vi "VisualizeLog.vi"() -> ()   [LabVIEW 2018, in "Visualization.lvlib" / "VisualizeStatus.lvclass"]
doc: "This VI opens the error log on file and displays all errors that have been logged to file."
uses:
  VisualizeStatus.lvclass
  VisualizeBase/VisualizeBase_class/Requests/clUserEventType.ctl
  <vilib>/event_ctls.llb/usereventprio.ctl
  <vilib>/Utility/error.llb/Error Cluster From Error Code.vi
  <vilib>/ErrorRing/Error Ring.xnode
  VisualizeBase/VisualizeBase_class/VisualizeBase.lvclass
  <userlib>/NIST/NISTErrorLib/NISTErrorLib.lvlib
panel:
  in  "btnClearFile":bool
  in  "btnClear":bool
  out "error out":errorcluster
  in  "File Path Control":path
  out "Status Message":string
  in  "btnRefresh":bool
  in  "QueName":string="ErrorLogVisQue"
  out "ErrorArray":errorcluster[](array[cluster])
  in  "btnStop":bool
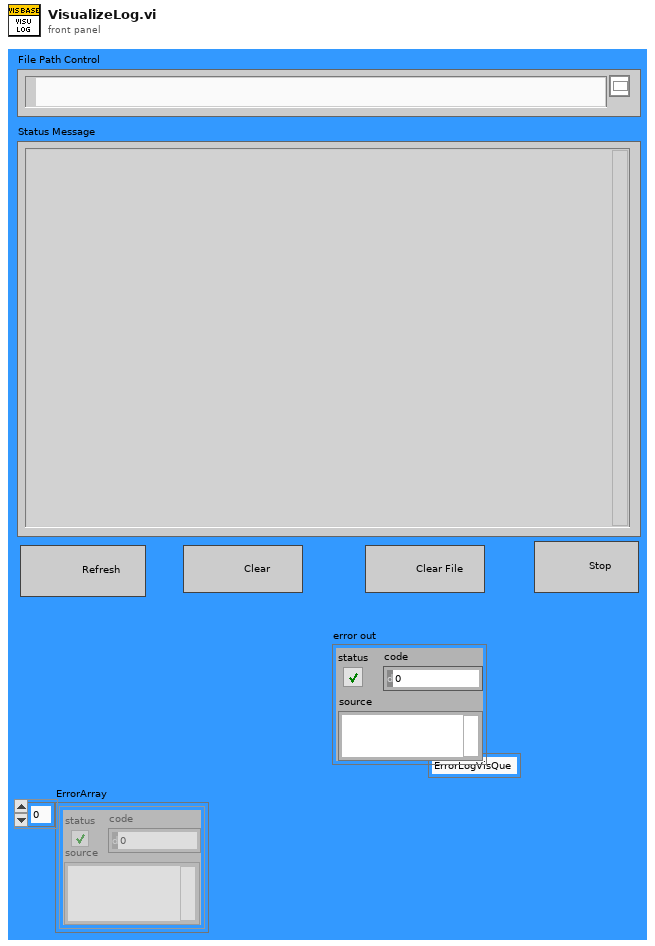
[diagram p1: front panel]
types:
  T1 = typedef "Visualization.lvlib/VisualizeBase.lvclass/clRequestEvents.ctl" = cluster{"StopRequest":refnum<user-event>, "ResetRequest":refnum<user-event>}
  T2 = enum16{"open", "replace", "create", "open or create", "replace or create", "replace or create with confirmation"}
  T3 = typedef "usereventprio.ctl" = enum32{"high priority", "normal priority"}
  T4 = typedef "Visualization.lvlib/VisualizeBase.lvclass/clUserEventType.ctl" = cluster{"BusIndex":i8, "Data":variant}
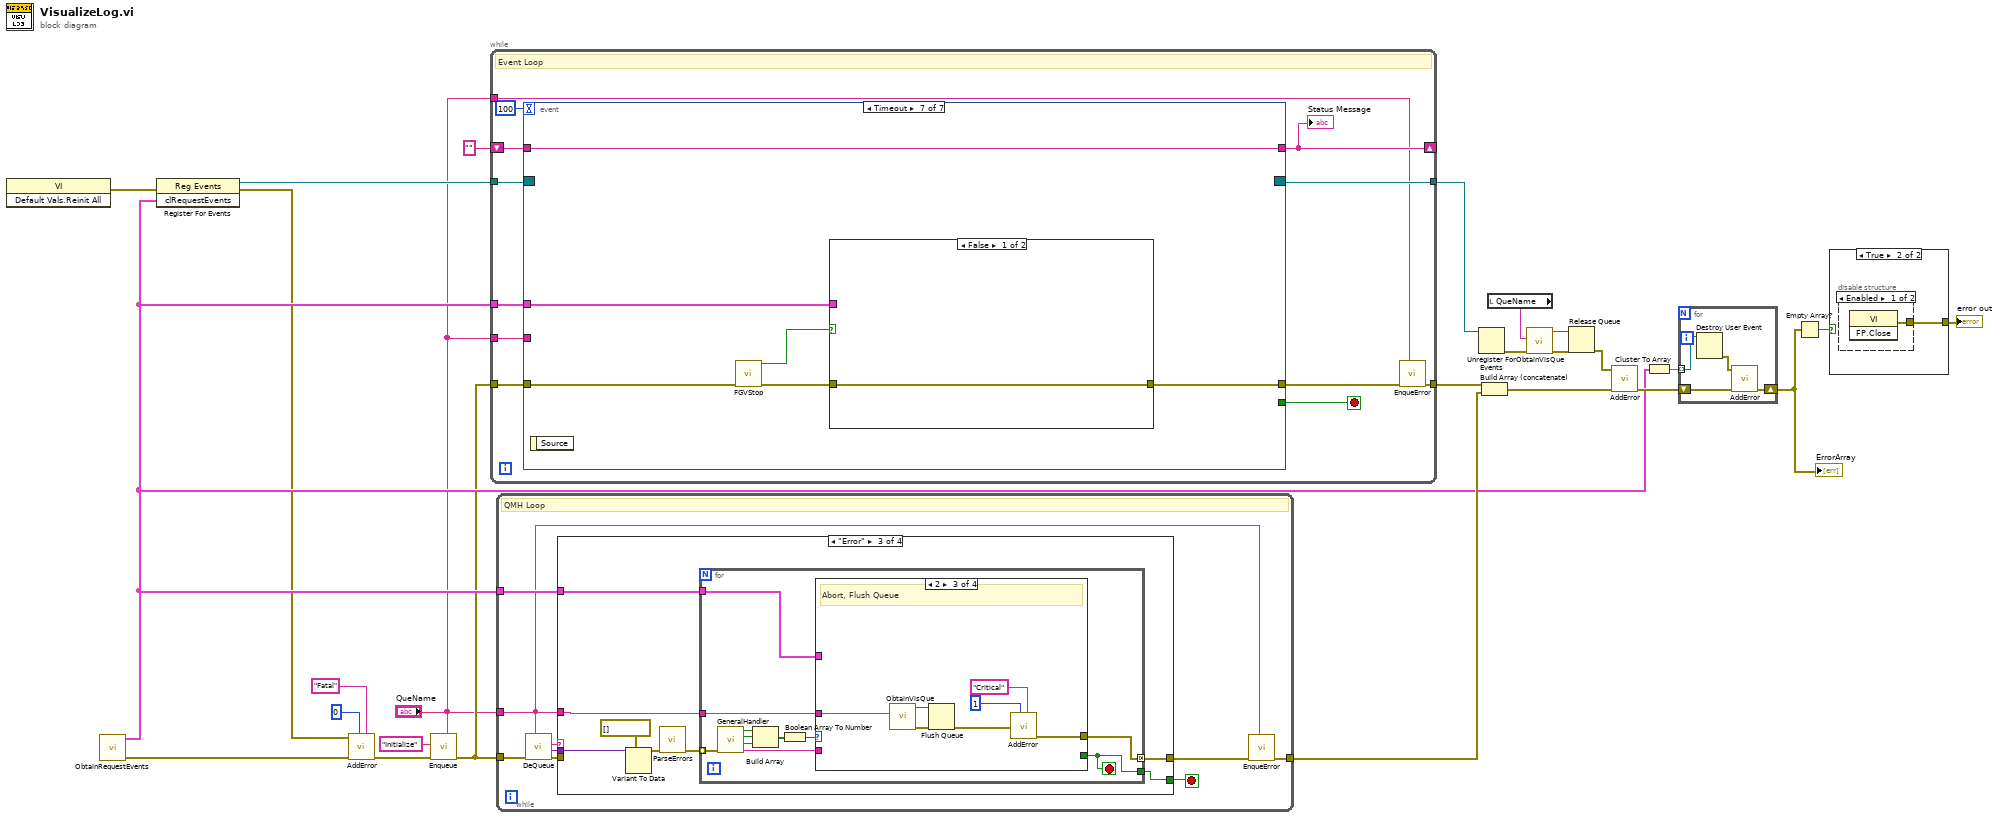
[diagram p0: block diagram]
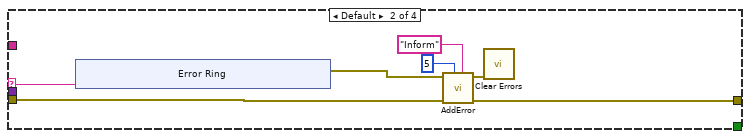
[diagram p3: hidden frame]
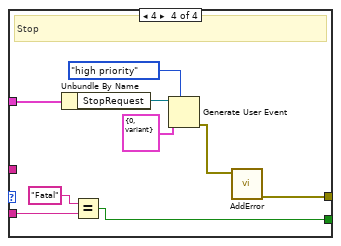
[diagram p6: hidden frame]
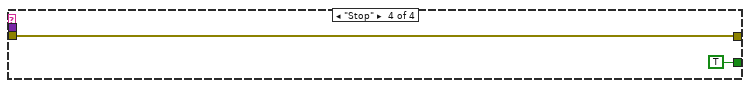
[diagram p7: hidden frame]
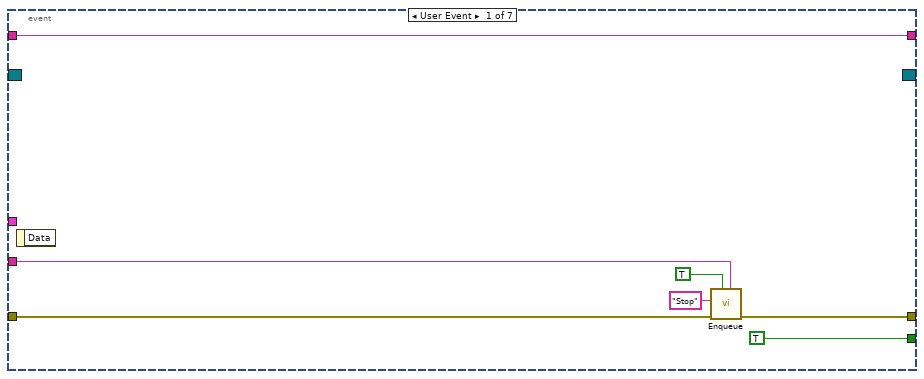
[diagram p8: hidden frame]
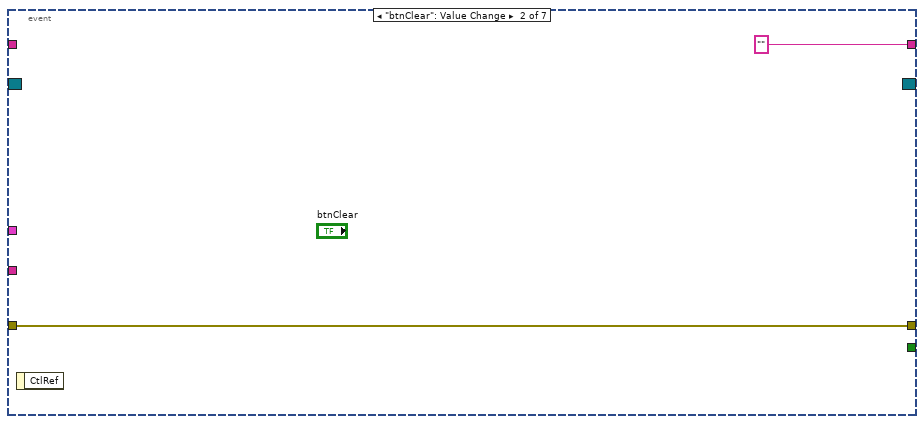
[diagram p9: hidden frame]
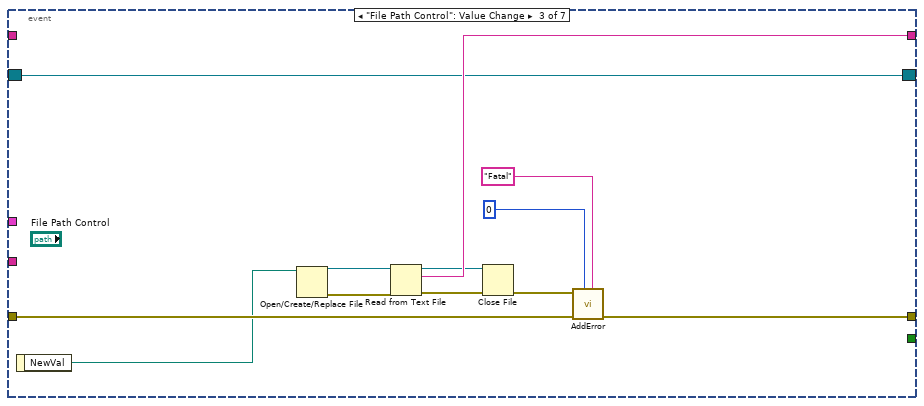
[diagram p10: hidden frame]
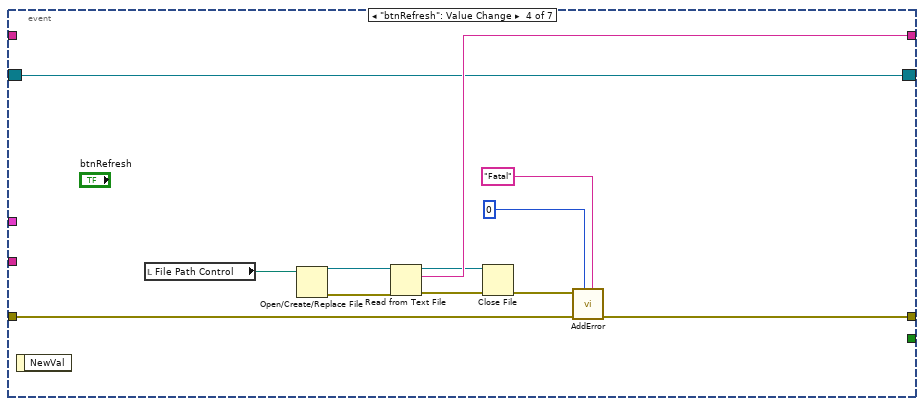
[diagram p11: hidden frame]
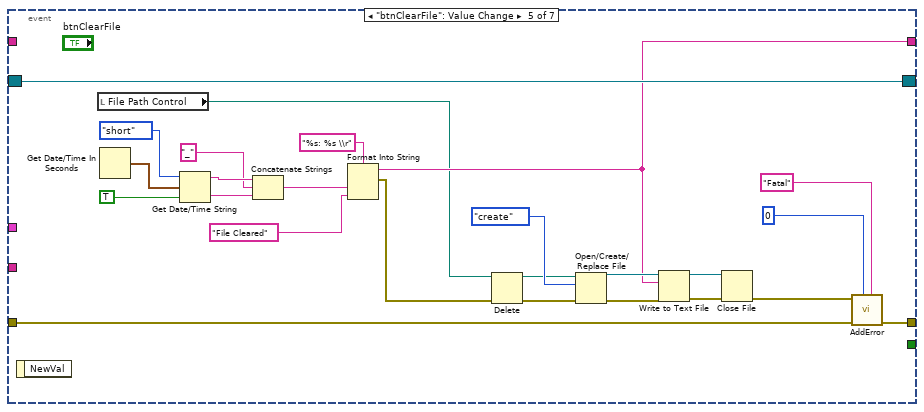
[diagram p12: hidden frame]
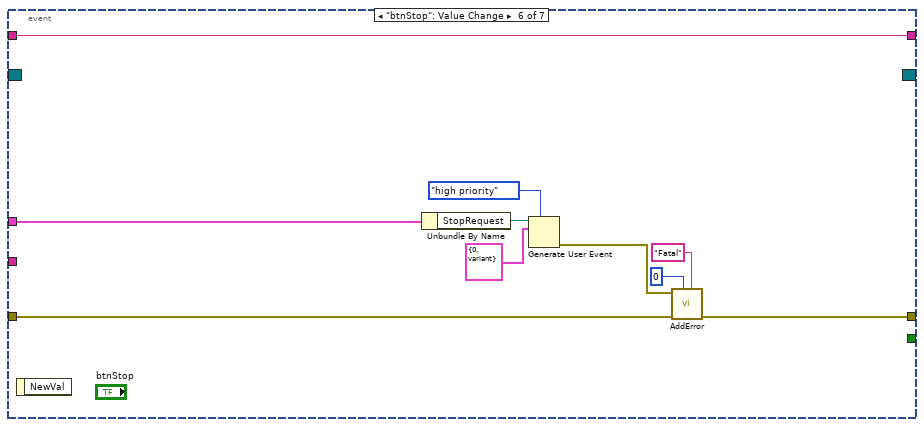
[diagram p13: hidden frame]
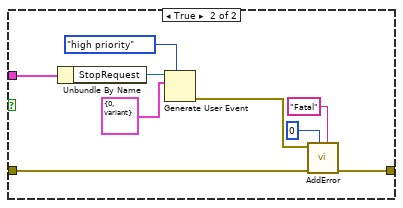
[diagram p14: hidden frame]
diagram:
  n1 = invoke class="VI" method="Default Vals.Reinit All"() -> (error out=w1:errorcluster)  [unwired: 3 in, 2 out]
  n2 = call "ObtainRequestEvents.vi"() -> ("Error"=w25:errorcluster[], "clRequestEvents"=w9:T1)  [unwired: 10 in]
  n3 = register-events(error in=w1, w9) -> (reference out=w10:refnum<event-registration>, error out=w8:errorcluster)  [unwired: 1 in]
  n4 = call <userlib>:"AddError.vi"("Severity"="Fatal", "Priority"=u8 0, "ErrorArray"=w25, "error in (no error)"=w8) -> ("ErrorArray"=w11:errorcluster[])  [unwired: 6 in, 1 out]
  n5 = call "Enqueue.vi"("QueName"="QueName", "Error"=w11, "Message"="Initialize") -> ("Error"=w7:errorcluster[])  [unwired: 8 in]
  n6 = while {
    tunnel: w10 -> [w38]
    tunnel: [w35] -> w22
    tunnel: [w34] -> w24
    tunnel: w9 -> [w33]
    shift-right: [w30] -> _
    shift-left: "" -> [w32]
    tunnel: w7 -> [w31]
    tunnel: "QueName" -> [w29]
    tunnel: "QueName" -> [w28]
    stop <- w37 stop-if-true
    # "Event Loop"
    n7 = event shown="[6] Timeout" {
      selector: w38 -> [_ _ w48 w61 w87 _ _]
      dyn-events: [_ _ w48 w61 w87 _ _] -> w34
      timeout: 100 -> [_ _ _ _ _ _ _]
      tunnel: [TRUE _ _ _ _ _ _] -> w37
      tunnel: [w44 w46 w53 w65 w91 w104 w112] -> w36
      tunnel: w33 -> [_ _ _ _ _ w99 w111]
      tunnel: [w39 "" w57 w69 w77 w97 w110] -> w30
      tunnel: w32 -> [w39 _ _ _ _ w97 w110]
      tunnel: w31 -> [w40 w46 w54 w66 w92 w98 w108]
      tunnel: w28 -> [w41 _ _ _ _ _ _]
      event User Event {
        n8 = event-data() -> ()  [unwired: 1 in, 1 out]
        n9 = call "Enqueue.vi"("QueName"=w41, "Priority? (F)"=TRUE, "Error"=w40, "Message"="Stop") -> ("Error"=w44:errorcluster[])  [unwired: 7 in]
      }
      event "btnClear": Value Change {
        n10 = event-data() -> ()  [unwired: 1 in, 1 out]
      }
      event "File Path Control": Value Change {
        n11 = event-data() -> ("NewVal"=w49:path)  [unwired: 1 in]
        n12 = Open/Create/Replace File(file path (use dialog)=w49) -> (refnum out=w58:refnum<file>, error out=w59:errorcluster)  [unwired: 5 in, 1 out]
        n13 = Read from Text File(file (use dialog)=w58, error in=w59) -> (refnum out=w55:refnum<file>, text=w57:string, error out=w56:errorcluster)  [unwired: 2 in, 1 out]
        n14 = Close File(refnum=w55, error in=w56) -> (error out=w52:errorcluster)  [unwired: 1 out]
        n15 = call <userlib>:"AddError.vi"("Severity"="Fatal", "Priority"=u8 0, "ErrorArray"=w54, "error in (no error)"=w52) -> ("ErrorArray"=w53:errorcluster[])  [unwired: 6 in, 1 out]
      }
      event "btnRefresh": Value Change {
        n16 = event-data() -> ()  [unwired: 1 in, 1 out]
        n17 = local read "File Path Control"() -> (w60:path)
        n18 = Open/Create/Replace File(file path (use dialog)=w60) -> (refnum out=w70:refnum<file>, error out=w71:errorcluster)  [unwired: 5 in, 1 out]
        n19 = Read from Text File(file (use dialog)=w70, error in=w71) -> (refnum out=w67:refnum<file>, text=w69:string, error out=w68:errorcluster)  [unwired: 2 in, 1 out]
        n20 = Close File(refnum=w67, error in=w68) -> (error out=w64:errorcluster)  [unwired: 1 out]
        n21 = call <userlib>:"AddError.vi"("Severity"="Fatal", "Priority"=u8 0, "ErrorArray"=w66, "error in (no error)"=w64) -> ("ErrorArray"=w65:errorcluster[])  [unwired: 6 in, 1 out]
      }
      event "btnClearFile": Value Change {
        n22 = event-data() -> ()  [unwired: 1 in, 1 out]
        n23 = local read "File Path Control"() -> (w75:path)
        n24 = Get Date/Time In Seconds() -> (seconds since 1Jan1904=w86:timestamp)
        n25 = Get Date/Time String(date format (0)=enum16{"short", "long", "abbreviated"}."short", seconds (now)=w86, want seconds? (F)=TRUE) -> (date string=w84:string, time string=w85:string)
        n26 = Concatenate Strings(w84, "_" ("string"), w85) -> (w83:string)
        n27 = Format Into String(format string="%s: %s \\r", w83, "File Cleared" ("Severity")) -> (resulting string=w77:string, error out=w74:errorcluster)  [unwired: 2 in]
        n28 = Delete(path (use dialog)=w75, error in=w74) -> (deleted path=w72:path, error out=w73:errorcluster)  [unwired: 3 in, 1 out]
        n29 = Open/Create/Replace File(file path (use dialog)=w72, error in=w73, operation (0:open)=T2."create") -> (refnum out=w95:refnum<file>, error out=w96:errorcluster)  [unwired: 3 in, 1 out]
        n30 = Write to Text File(file (use dialog)=w95, text=w77, error in=w96) -> (refnum out=w93:refnum<file>, error out=w94:errorcluster)  [unwired: 1 in, 1 out]
        n31 = Close File(refnum=w93, error in=w94) -> (error out=w90:errorcluster)  [unwired: 1 out]
        n32 = call <userlib>:"AddError.vi"("Severity"="Fatal", "Priority"=u8 0, "ErrorArray"=w92, "error in (no error)"=w90) -> ("ErrorArray"=w91:errorcluster[])  [unwired: 6 in, 1 out]
      }
      event "btnStop": Value Change {
        n33 = event-data() -> ()  [unwired: 1 in, 1 out]
        n34 = Unbundle By Name(w99) -> ("StopRequest"=w105:refnum<user-event>)
        n35 = Generate User Event(priority (normal)=usereventprio."high priority", user event=w105, event data cluster=T4 {"BusIndex"=0, "Data"=variant} ("event data")) -> (error out=w106:errorcluster)  [unwired: 1 in, 1 out]
        n36 = call <userlib>:"AddError.vi"("Severity"="Fatal" ("String"), "Priority"=u8 0, "ErrorArray"=w98, "error in (no error)"=w106) -> ("ErrorArray"=w104:errorcluster[])  [unwired: 6 in, 1 out]
      }
      event Timeout {
        n37 = event-data() -> ()  [unwired: 1 in, 1 out]
        n38 = call "FGVStop.vi"("Error In"=w108) -> ("Error Out"=w107:errorcluster[], "Value"=w109:bool)  [unwired: 9 in]
        n39 = case shown="False" w109 {
          tunnel: [w113 w120] -> w112
          tunnel: w111 -> [_ w115]
          tunnel: w107 -> [w113 w114]
          frame False {
          }
          frame True {
            n40 = Unbundle By Name(w115) -> ("StopRequest"=w121:refnum<user-event>)
            n41 = Generate User Event(priority (normal)=usereventprio."high priority", user event=w121, event data cluster=T4 {"BusIndex"=0, "Data"=variant} ("event data")) -> (error out=w122:errorcluster)  [unwired: 1 in, 1 out]
            n42 = call <userlib>:"AddError.vi"("Severity"="Fatal" ("String"), "Priority"=u8 0, "ErrorArray"=w114, "error in (no error)"=w122) -> ("ErrorArray"=w120:errorcluster[])  [unwired: 6 in, 1 out]
          }
        }
      }
    }
    "Status Message" <- w30
    n43 = call "EnqueError.vi"("QueName"=w29, "Error"=w36) -> ("Error"=w35:errorcluster[])  [unwired: 9 in]
  }
  n44 = while {
    tunnel: w7 -> [w131]
    tunnel: [w125] -> w21
    tunnel: w9 -> [w124]
    tunnel: "QueName" -> [w123]
    stop <- w126 stop-if-true
    # "QMH Loop"
    n45 = call "DeQueue.vi"("QueName"=w123, "Error"=w131) -> ("Error"=w128:errorcluster[], "Data"=w129:variant, "Message"=w130:string)  [unwired: 7 in]
    n46 = case shown="\"Error\"" w130 {
      selector: w130 -> [_ w139 _ _]
      tunnel: w129 -> [_ _ w154 _]
      tunnel: w128 -> [w132 w137 _ w182]
      tunnel: [w132 w136 w150 w182] -> w127
      tunnel: [_ _ w149 TRUE] -> w126
      tunnel: w124 -> [_ _ w148 _]
      tunnel: w123 -> [_ _ w147 _]
      frame "Initialize" {
      }
      frame Default {
        n47 = xnode "Error Ring"("parameter 0"=w139) -> ("error out"=w138:errorcluster)
        n48 = call <userlib>:"AddError.vi"("Severity"="Inform" ("String"), "Priority"=u8 5, "ErrorArray"=w137, "error in (no error)"=w138) -> ("ErrorArray"=w136:errorcluster[], "error out"=w135:errorcluster)  [unwired: 6 in]
        n49 = call <vilib>:"Clear Errors.vi"("error in (no error)"=w135) -> ()  [unwired: 5 in, 2 out]
      }
      frame "Error" {
        n50 = Variant To Data(type=errorcluster[] [], Variant=w154) -> (data=w152:errorcluster[])  [unwired: 1 in, 1 out]
        n51 = call <userlib>:"ParseErrors.vi"("ErrorArray"=w152) -> ("ErrorArray"=w151:errorcluster[])  [unwired: 8 in, 2 out]
        n52 = for {
          tunnel: w151 -> [w165] mode=indexing
          tunnel: [w159] -> w150 mode=concatenating
          tunnel: [w157] -> w149
          tunnel: w148 -> [w156]
          tunnel: w147 -> [w155]
          stop <- w157 stop-if-true
          n53 = call <userlib>:"GeneralHandler.vi"("error in (no error)"=w165) -> ("Severity"=w158:string, "Stop"=w162:bool, "Abort"=w163:bool, "Continue"=w164:bool)  [unwired: 6 in, 1 out]
          n54 = Build Array(w164, w163, w162) -> (w161:bool[])
          n55 = Boolean Array To Number(Boolean array=w161) -> (number=w160:u32)
          n56 = case shown="2" w160 {
            tunnel: [_ _ w170 w180] -> w159
            tunnel: w158 -> [_ _ _ w176]
            tunnel: [_ _ _ w174] -> w157
            tunnel: w156 -> [_ _ _ w173]
            tunnel: w155 -> [_ _ w166 _]
            frame 0, Default {
              # "No Dialog"
            }
            frame 1 {
              # "Continue"
            }
            frame 2 {
              # "Abort, Flush Queue"
              n57 = call "ObtainVisQue.vi"("QueName"=w166) -> ("error out"=w172:errorcluster, "queue out"=w171:refnum<queue>)  [unwired: 9 in]
              n58 = Flush Queue(queue=w171, error in (no error)=w172) -> (error out=w169:errorcluster)  [unwired: 2 out]
              n59 = call <userlib>:"AddError.vi"("Severity"="Critical" ("String"), "Priority"=u8 1, "error in (no error)"=w169) -> ("ErrorArray"=w170:errorcluster[])  [unwired: 7 in, 1 out]
            }
            frame 4 {
              # "Stop"
              n60 = Unbundle By Name(w173) -> ("StopRequest"=w181:refnum<user-event>)
              n61 = Equal?(x="Fatal", y=w176) -> (x = y?=w174:bool)
              n62 = Generate User Event(priority (normal)=usereventprio."high priority", user event=w181, event data cluster=T4 {"BusIndex"=0, "Data"=variant} ("event data")) -> (error out=w179:errorcluster)  [unwired: 1 in, 1 out]
              n63 = call <userlib>:"AddError.vi"("error in (no error)"=w179) -> ("ErrorArray"=w180:errorcluster[])  [unwired: 9 in, 1 out]
            }
          }
        }
      }
      frame "Stop" {
      }
    }
    n64 = call "EnqueError.vi"("QueName"=w123, "Error"=w127) -> ("Error"=w125:errorcluster[])  [unwired: 9 in]
  }
  n65 = Unregister For Events(event registration refnum=w24) -> (error out=w20:errorcluster)  [unwired: 1 in]
  n66 = Build Array (concatenate)(w22, w21) -> (w18:errorcluster[])
  n67 = local read "QueName"() -> (w19:string)
  n68 = call "ObtainVisQue.vi"("error in (no error)"=w20, "QueName"=w19) -> ("error out"=w17:errorcluster, "queue out"=w16:refnum<queue>)  [unwired: 8 in]
  n69 = Release Queue(queue=w16, error in (no error)=w17) -> (error out=w15:errorcluster)  [unwired: 1 in, 2 out]
  n70 = call <userlib>:"AddError.vi"("ErrorArray"=w18, "error in (no error)"=w15) -> ("ErrorArray"=w14:errorcluster[])  [unwired: 8 in, 1 out]
  n71 = Cluster To Array(cluster=w9) -> (array=w23:refnum<user-event>[])
  n72 = for {
    tunnel: w23 -> [w187] mode=indexing
    shift-right: [w186] -> w13
    shift-left: w14 -> [w185]
    n73 = Destroy User Event(user event=w187) -> (error out=w184:errorcluster)  [unwired: 1 in]
    n74 = call <userlib>:"AddError.vi"("ErrorArray"=w185, "error in (no error)"=w184) -> ("ErrorArray"=w186:errorcluster[])  [unwired: 8 in, 1 out]
  }
  "ErrorArray" <- w13
  n75 = Empty Array?(array=w13) -> (empty?=w12:bool)
  n76 = case shown="True" w12 {
    tunnel: [_ w188] -> w2
    frame False {
    }
    frame True {
      n77 = disable-structure shown="Enabled" {
        disable-tunnel: [w189 _] -> w188
        frame Enabled {
          n78 = invoke class="VI" method="FP.Close"() -> (error out=w189:errorcluster)  [unwired: 3 in, 2 out]
        }
        frame Disabled {
        }
      }
    }
  }
  "error out" <- w2
